vi "MultiBiasScanCurrent.vi"() -> ()   [LabVIEW 2014]
uses:
  <userlib>/Nanonis Prog Interface V5/Nanonis Prog Interface.lvlib
panel:
  in  "Settling time (s)":dbl=0.7 format="%#_6p"
  in  "img bias":bool=TRUE
  in  "img bias":dbl=-0.0012 format="%#_6p"
  in  "img delay (s)":u32
  out "tipLift":dbl=1e-10 format="%#_6p"
  in  "TipLiftList":i32(listbox)
  in  "Const Height":bool=TRUE
  in  "Positions":bool
  in  "Center coordinates (m)":cluster{"Xc":sgl, "Yc":sgl}={"Xc"=nan, "Yc"=nan} {"Yc" format="%.2p"; "Xc" format="%.2p"}
  in  "Size (m)":cluster{"Width":sgl, "Height":sgl}={"Width"=nan, "Height"=nan} caption="Size (m) (NaN=no change)" {"Height" format="%.2p"; "Width" format="%.2p"}
  in  "Numeric":i32
  in  "PositionList":i32(listbox)
  in  "CurrentList":i32(listbox)
  in  "BiasList":i32(listbox)
  out "Current":dbl=2.5e-11 format="%#_6p"
  out "Bias":dbl=0.02 format="%#_6p"
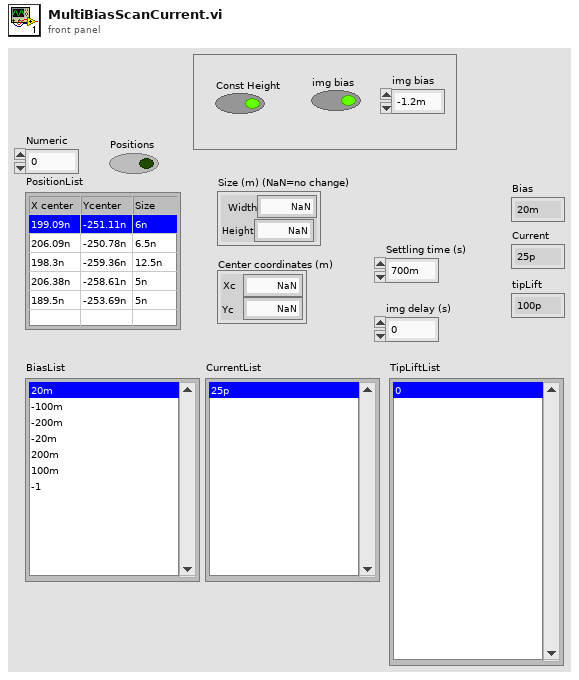
[diagram p1: front panel]
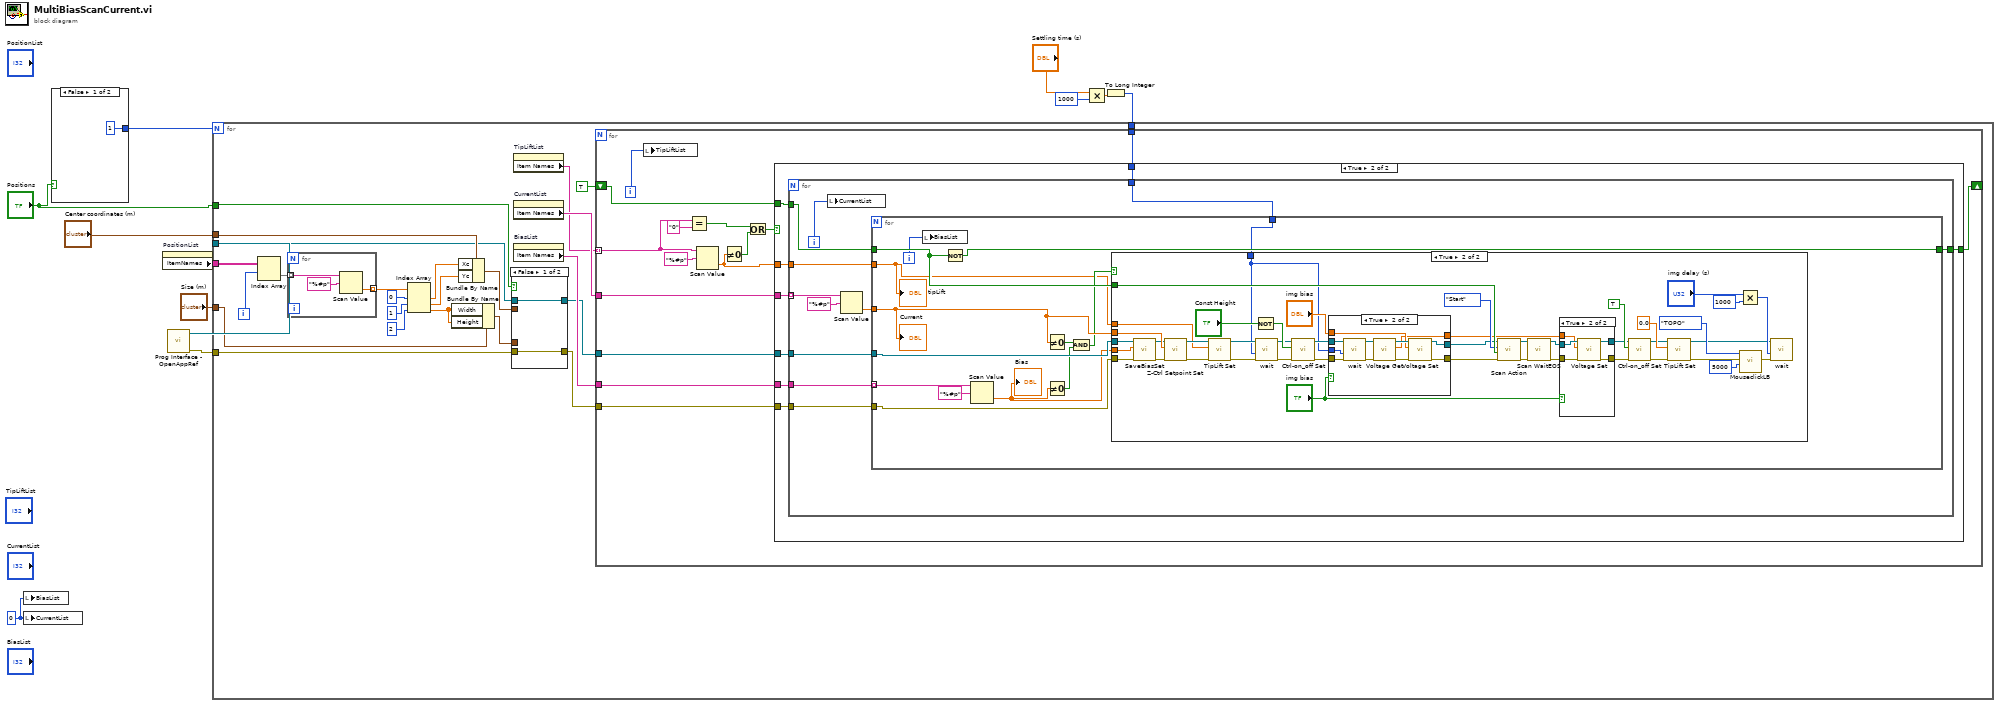
[diagram p0: block diagram]
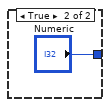
[diagram p2: hidden frame]
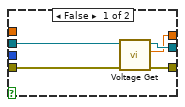
[diagram p6: hidden frame]
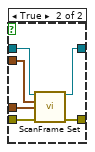
[diagram p7: hidden frame]
diagram:
  w12 = 0 ("BiasList")
  n1 = local write "BiasList"(w12) -> ()
  n2 = local write "CurrentList"(w12) -> ()
  n3 = case shown="False" "Positions" {
    tunnel: [1 ("Numeric") "Numeric"] -> w9
    frame False {
    }
    frame True {
    }
  }
  n4 = property on="PositionList" class="MCListbox (strict)"() -> ("ItemNames"=w8:string[][])  [unwired: 2 in, 2 out]
  n5 = call <userlib>:"Prog Interface - OpenAppRef.vi"() -> ("Error out"=w10:errorcluster, "Application reference"=w11:refnum<vi>)  [unwired: 6 in]
  n6 = Multiply(x="Settling time (s)", y=u32 1000) -> (x*y=w1:dbl)
  n7 = To Long Integer(number=w1) -> (32bit integer=w2:i32)
  n8 = for {
    N: w9 -> [_]
    tunnel: w11 -> [w27]
    tunnel: w10 -> [w26]
    tunnel: w8 -> [w35]
    tunnel: "Size (m)" -> [w32]
    tunnel: "Center coordinates (m)" -> [w30]
    tunnel: "Positions" -> [w17]
    tunnel: w2 -> [w15]
    i -> [w34]
    n9 = Index Array(array=w35, index (row)=w34) -> (element=w33:string[])  [unwired: 1 in]
    n10 = for {
      tunnel: w33 -> [w163] mode=indexing
      tunnel: [w162] -> w31 mode=indexing
      n11 = Scan Value(string=w163, format string="%#p") -> (value=w162:dbl)  [unwired: 1 in, 1 out]
    }
    n12 = Index Array(array=w31, index #1=0 ("index"), index #2=1 ("index"), index #3=2 ("index")) -> (element #1=w20:dbl, element #2=w19:dbl, element #3=w18:dbl)
    n13 = Bundle By Name(cluster=w32, "Width"=w18, "Height"=w18) -> (w29:cluster{"Width":sgl, "Height":sgl})
    n14 = Bundle By Name(cluster=w30, "Xc"=w20, "Yc"=w19) -> (w28:cluster{"Xc":sgl, "Yc":sgl})
    n15 = case shown="False" w17 {
      tunnel: w29 -> [_ w161]
      tunnel: w28 -> [_ w160]
      tunnel: w27 -> [w155 w159]
      tunnel: w26 -> [w154 w158]
      tunnel: [w155 w157] -> w25
      tunnel: [w154 w156] -> w24
      frame False {
      }
      frame True {
        n16 = call <userlib>:"ScanFrame Set.vi"("Application ref in"=w159, "Center coordinates (m)"=w160, "Size (m)"=w161, "error in (no error)"=w158) -> ("Application ref out"=w157:refnum<vi>, "error out"=w156:errorcluster)  [unwired: 10 in]
      }
    }
    n17 = property on="TipLiftList" class="LstBox (strict)"() -> ("Item Names"=w16:string[])  [unwired: 2 in, 2 out]
    n18 = property on="CurrentList" class="LstBox (strict)"() -> ("Item Names"=w36:string[])  [unwired: 2 in, 2 out]
    n19 = property on="BiasList" class="LstBox (strict)"() -> ("Item Names"=w37:string[])  [unwired: 2 in, 2 out]
    n20 = for {
      tunnel: w37 -> [w52]
      tunnel: w36 -> [w51]
      tunnel: w25 -> [w50]
      tunnel: w24 -> [w49]
      tunnel: w16 -> [w46] mode=indexing
      shift-right: [w40] -> _
      shift-left: TRUE ("Direction: up/down (T=up)") -> [w53]
      tunnel: w15 -> [w39]
      i -> [w47]
      n21 = local write "TipLiftList"(w47) -> ()
      n22 = Equal?(x=w46, y="0") -> (x = y?=w41:bool)
      n23 = Scan Value(string=w46, format string="%#p") -> (value=w45:dbl)  [unwired: 1 in, 1 out]
      n24 = Not Equal To 0?(x=w45) -> (x != 0?=w44:bool)
      n25 = Or(x=w41, y=w44) -> (x .or. y?=w43:bool)
      n26 = case shown="True" w43 {
        tunnel: w53 -> [w54 w62]
        tunnel: w52 -> [_ w61]
        tunnel: w51 -> [_ w60]
        tunnel: w50 -> [_ w59]
        tunnel: w49 -> [_ w58]
        tunnel: w45 -> [_ w57]
        tunnel: [w54 w56] -> w40
        tunnel: w39 -> [_ w55]
        frame False {
        }
        frame True {
          n27 = for {
            tunnel: w62 -> [w73]
            tunnel: w59 -> [w72]
            tunnel: w58 -> [w71]
            tunnel: w61 -> [w70]
            tunnel: w60 -> [w68] mode=indexing
            tunnel: w57 -> [w65]
            tunnel: [w64] -> w56
            tunnel: w55 -> [w63]
            i -> [w66]
            n28 = local write "CurrentList"(w66) -> ()
            n29 = Scan Value(string=w68, format string="%#p") -> (value=w67:dbl)  [unwired: 1 in, 1 out]
            n30 = for {
              tunnel: w70 -> [w82] mode=indexing
              tunnel: w72 -> [w84]
              tunnel: w71 -> [w83]
              tunnel: w67 -> [w78]
              tunnel: w65 -> [w75]
              tunnel: w73 -> [w86]
              tunnel: [w85] -> w64
              tunnel: w63 -> [w74]
              i -> [w76]
              n31 = local write "BiasList"(w76) -> ()
              n32 = Not(x=w86) -> (.not. x?=w85:bool)
              n33 = Scan Value(string=w82, format string="%#p") -> (value=w79:dbl)  [unwired: 1 in, 1 out]
              "Bias" <- w79
              n34 = Not Equal To 0?(x=w78) -> (x != 0?=w81:bool)
              n35 = Not Equal To 0?(x=w79) -> (x != 0?=w80:bool)
              n36 = Compound Arithmetic op=AND(w81, w80) -> (w77:bool)
              n37 = case shown="True" w77 {
                tunnel: w86 -> [_ w119]
                tunnel: w79 -> [_ w125]
                tunnel: w84 -> [_ w129]
                tunnel: w83 -> [_ w126]
                tunnel: w78 -> [_ w130]
                tunnel: w75 -> [_ w114]
                tunnel: w74 -> [_ w88]
                frame False {
                }
                frame True {
                  n38 = call "SaveBiasSet.vi"("Application ref in"=w129, "Bias (V)"=w125, "error in (no error)"=w126) -> ("Application ref out"=w128:refnum<vi>, "Error out"=w127:errorcluster)  [unwired: 6 in]
                  n39 = call <userlib>:"Z-Ctrl Setpoint Set.vi"("error in (no error)"=w127, "Z Controller setpoint"=w130, "Application ref in"=w128) -> ("error out"=w115:errorcluster, "Application ref out"=w117:refnum<vi>)  [unwired: 7 in]
                  n40 = call <userlib>:"TipLift Set.vi"("error in (no error)"=w115, "TipLift (m)"=w114, "Application ref in"=w117) -> ("error out"=w89:errorcluster, "Application ref out"=w116:refnum<vi>)  [unwired: 7 in]
                  n41 = Not(x="Const Height") -> (.not. x?=w121:bool)
                  n42 = call "wait.vi"("error in"=w89, "milliseconds to wait"=w88, "application reference in"=w116) -> ("error out"=w90:errorcluster, "application reference out"=w91:refnum<vi>)  [unwired: 7 in]
                  n43 = call <userlib>:"Ctrl-on_off Set.vi"("error in (no error)"=w90, "Z Controller ON/OFF"=w121, "Application ref in"=w91) -> ("error out"=w109:errorcluster, "Application ref out"=w111:refnum<vi>)  [unwired: 7 in]
                  n44 = case shown="True" "img bias" {
                    tunnel: w111 -> [w142 w144]
                    tunnel: [w141 w151] -> w110
                    tunnel: w109 -> [w138 w147]
                    tunnel: [w139 w150] -> w108
                    tunnel: "img bias" -> [_ w149]
                    tunnel: [w140 w148] -> w105
                    tunnel: w88 -> [_ w143]
                    frame False {
                      n45 = call <userlib>:"Voltage Get.vi"("error in (no error)"=w138, "Application ref in"=w142) -> ("error out"=w139:errorcluster, "Bias (V)"=w140:sgl, "Application ref out"=w141:refnum<vi>)  [unwired: 7 in]
                    }
                    frame True {
                      n46 = call "wait.vi"("error in"=w147, "milliseconds to wait"=w143, "application reference in"=w144) -> ("error out"=w146:errorcluster, "application reference out"=w145:refnum<vi>)  [unwired: 7 in]
                      n47 = call <userlib>:"Voltage Get.vi"("error in (no error)"=w146, "Application ref in"=w145) -> ("error out"=w153:errorcluster, "Bias (V)"=w148:sgl, "Application ref out"=w152:refnum<vi>)  [unwired: 7 in]
                      n48 = call <userlib>:"Voltage Set.vi"("Error in (no error)"=w153, "Bias (V)"=w149, "Application ref in"=w152) -> ("Error out"=w150:errorcluster, "Application ref out"=w151:refnum<vi>)  [unwired: 7 in]
                    }
                  }
                  n49 = call <userlib>:"Scan Action.vi"("error in (no error)"=w108, "Direction: up/down (T=up)"=w119, "Scan action (Start)"=enum16{"Start", "Stop", "Pause", "Resume"}."Start", "Application ref in"=w110) -> ("error out"=w124:errorcluster, "Application ref out"=w123:refnum<vi>)  [unwired: 5 in]
                  n50 = call <userlib>:"Scan WaitEOS.vi"("error in (no error)"=w124, "Application ref in"=w123) -> ("error out"=w103:errorcluster, "Application ref out"=w104:refnum<vi>)  [unwired: 5 in, 2 out]
                  n51 = case shown="True" "img bias" {
                    tunnel: w104 -> [w132 w135]
                    tunnel: [w132 w137] -> w102
                    tunnel: [w131 w136] -> w101
                    tunnel: w103 -> [w131 w134]
                    tunnel: w105 -> [_ w133]
                    frame False {
                    }
                    frame True {
                      n52 = call <userlib>:"Voltage Set.vi"("Error in (no error)"=w134, "Bias (V)"=w133, "Application ref in"=w135) -> ("Error out"=w136:errorcluster, "Application ref out"=w137:refnum<vi>)  [unwired: 7 in]
                    }
                  }
                  n53 = call <userlib>:"Ctrl-on_off Set.vi"("error in (no error)"=w101, "Z Controller ON/OFF"=TRUE, "Application ref in"=w102) -> ("error out"=w100:errorcluster, "Application ref out"=w99:refnum<vi>)  [unwired: 7 in]
                  n54 = call <userlib>:"TipLift Set.vi"("error in (no error)"=w100, "TipLift (m)"=sgl 0.0, "Application ref in"=w99) -> ("error out"=w113:errorcluster, "Application ref out"=w92:refnum<vi>)  [unwired: 7 in]
                  n55 = Multiply(x="img delay (s)", y=u32 1000) -> (x*y=w94:u32)
                  n56 = call "MouseclickLB.vi"("nMilliseconds"=5000, "error in (no error)"=w113, "Click"=enum16{"Header", "TOPO", "STS", "GRID"}."TOPO") -> ("error out"=w93:errorcluster)  [unwired: 8 in]
                  n57 = call "wait.vi"("error in"=w93, "milliseconds to wait"=w94, "application reference in"=w92) -> ()  [unwired: 7 in, 2 out]
                }
              }
              "Current" <- w78
              "tipLift" <- w75
            }
          }
        }
      }
    }
  }
